vi "MTDC_Prototype.vi"() -> ()   [LabVIEW 2025]
uses:
  Desktop/STM-Auto-Project/QMH CTLS/Scan_Params (QMH).ctl
  <instrlib>/SMS LabVIEW Drivers/Source Code/Public/PSU Status.ctl
  Desktop/STM-Auto-Project/QMH CTLS/Sweeper.ctl
  <instrlib>/SMS LabVIEW Drivers/Source Code/Cryogenic Ltd SMSXXX.lvlib
  Downloads/OneDrive_2025-09-03/Instrument Controls/Temp Cntrl.ctl
  Desktop/Magnetic Drift Correction/XY_Coords(Final).ctl
panel:
  out "Translation (m)":T1
  out "Final coordinates (m)":cluster{"Xc":sgl, "Yc":sgl} {"Yc" format="%.4p"; "Xc" format="%.4p"}
  out "Initial coordinates (m)":cluster{"Xc":sgl, "Yc":sgl} {"Yc" format="%.4p"; "Xc" format="%.4p"}
  out "Temp. Array":dbl[](array[numeric])
  out "Current Temp":dbl format="%#.5f"
  out "Current MID (T)":dbl
  out "Output (T)":dbl
  in  "P-Mode Ramp Rate (A/s)":dbl=0.02
  out "Initial MID (T)":dbl
  in  "Serial Configuration":T2={"Baud Rate"=57600, "Parity"=1, "Data Bits"=7, "Stop Bits"=10, "Flow Control"=0}
  in  "Field and Temp Range":T3={"VISA (Magnet)"="COM4", "Fields(T)"=[], "Temps(K)"=[], "VISA (Temp) "="COM1", "Port number (3364)"=3364}
  in  "Lead- Mode Ramp Rate (A/s)":dbl=0.02
  out "Errors":errorcluster[](array[cluster])
  out "Current Index":i32
  in  "stop":bool
  in  "Start":bool
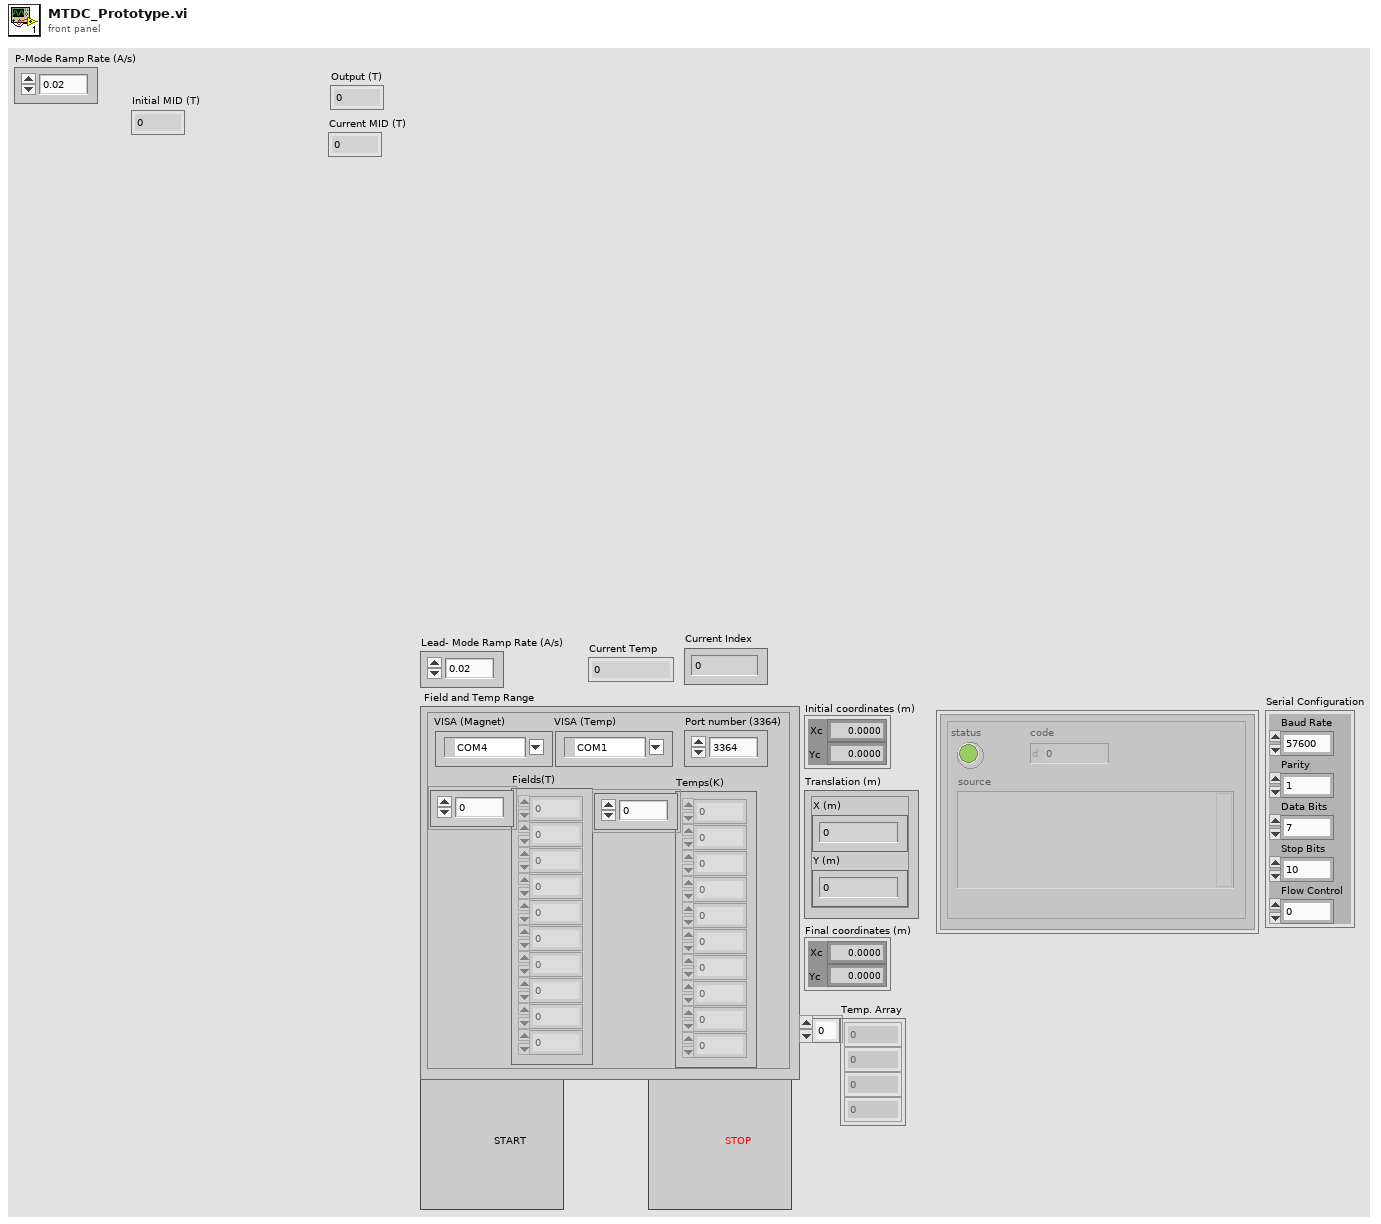
[diagram p1: front panel]
types:
  T1 = typedef "XY_Coords(Final).ctl" = cluster{"X (m)":dbl, "Y (m)":dbl}
  T2 = cluster{"Baud Rate":u32, "Parity":u16, "Data Bits":u16, "Stop Bits":u16, "Flow Control":u16}
  T3 = cluster{"VISA (Magnet)":refnum<visa-resource-name>, "Fields(T)":dbl[], "Temps(K)":dbl[], "VISA (Temp) ":refnum<visa-resource-name>, "Port number (3364)":u32}
  T4 = enum16{"1. INIT MAG", "2. MAG ON", "3. MAG_STAB", "4. MAG IDLE", "5. PREP NEXT FIELD", "6. APPLY NEXT FIELD", "7. PREP OFF", "8. MAG OFF (Reset)"}
  T5 = enum16{"1. BIAS", "2. INIT_SCAN", "3. SCAN_IDLE", "4. INTER_SCAN", "5. NEW_COORDS_&_FRAME", "6. FINAL_SCAN", "7. POLL BIAS ", "8. Z-CONT.", "9. STOP"}
  T6 = typedef "Temp Cntrl.ctl" = cluster{"Range (0:Off)":u16, "Manual Output (0.00 %)":dbl, "Rate (D) (0.0 %)":dbl, "Reset (I) (20.0)":dbl, "Gain (P) (50.0)":dbl, "Power Up Enable (F: Disable)":bool, "Max User Current (2.000)":dbl, "Heater Resistance (1:25 Ohms)":u16, "Max Current (0:User Specified)":u16, "Heater Out Display (1:Current)":u16, "Mode (0:Off)":u16, "Input (0:None)":u16, "Target Temp (K)":dbl, "Serial Configuration":cluster{"Baud Rate":u32, "Parity":u16, "Data Bits":u16, "Stop Bits":u16, "Flow Control":u16}, "VISA resource name":refnum<visa-resource-name>, "Configure Control Parameters (0: Configure)":u16, "Enable Setpoint (F:Disable)":bool, "Input (0:A)":u16, "Data Source (0:Kelvin)":u16, "Output's Control Loop (1:1)":u16, "STND DEV Threshold ":dbl, "Mean Tolerance ":dbl, "Current State":enum16{"1. INIT TEMP", "2. TC ON", "3. POLL_TEMPS", "4. TEMP_STAB", "5. TC IDLE", "6. APPLY NEXT TEMP", "7. TC OFF (Reset)"}}
  T7 = enum16{"NO CHANGE", "SET TEMP & FIELD", "SWEEP IDLE", "NEXT TEMP & FIELD", "SWEEP DONE"}
  T8 = typedef "Sweeper.ctl" = cluster{"Temps(K)":dbl[], "Fields(T)":dbl[], "Sweep States":enum16{"NO CHANGE", "SET TEMP & FIELD", "SWEEP IDLE", "NEXT TEMP & FIELD", "SWEEP DONE"}}
  T9 = enum16{"1. INIT TEMP", "2. TC ON", "3. POLL_TEMPS", "4. TEMP_STAB", "5. TC IDLE", "6. APPLY NEXT TEMP", "7. TC OFF (Reset)"}
  T10 = typedef "PSU Status.ctl" = cluster{"Ramp Target":enum16{"ZERO", "MID", "MAX"}, "Pause":bool, "Switch Heater":bool, "Persistent Field":dbl, "Persistent Current":dbl, "Tesla":bool, "Output (T)":dbl, "Output (A)":dbl, "X Trip":enum16{"DISABLED", "ENABLED", "ACTIVE"}, "Ramp Rate (A/s)":dbl, "V Limit (V)":dbl, "Heater Voltage":dbl, "MAX Setpoint (A)":dbl, "MAX Setpoint (T)":dbl, "MID Setpoint (A)":dbl, "MID Setpoint (T)":dbl, "Lock":bool, "Field Constant":dbl, "Remote":bool, "Direction":enum16{"POSITIVE", "NEGATIVE", "OPEN", "UNIPOLAR"}, "Helium Level":u16, "Quench !":bool, "Voltage":dbl, "V Limit !":bool, "Ramping":bool, "At Target":bool, "Trip Field":dbl, "Trip Current":dbl, "Current State":enum16{"1. INIT MAG", "2. MAG ON", "3. MAG_STAB", "4. MAG IDLE", "5. PREP NEXT FIELD", "6. APPLY NEXT FIELD", "7. PREP OFF", "8. MAG OFF (Reset)"}, "MAG Reference":refnum<visa-resource-name>}
  T11 = typedef "Scan_Params (QMH).ctl" = cluster{"Setpoint (I)":dbl[], "Bias (V)":dbl[], "Number of scans":u8, "Port number (3364)":u32, "Avoid zero threshold (V)":dbl, "Current State":enum16{"1. BIAS", "2. INIT_SCAN", "3. SCAN_IDLE", "4. INTER_SCAN", "5. NEW_COORDS_&_FRAME", "6. FINAL_SCAN", "7. POLL BIAS ", "8. Z-CONT.", "9. STOP"}}
  T12 = enum16{"RAMP TO ZERO", "RAMP TO MID", "RAMP TO MAX"}
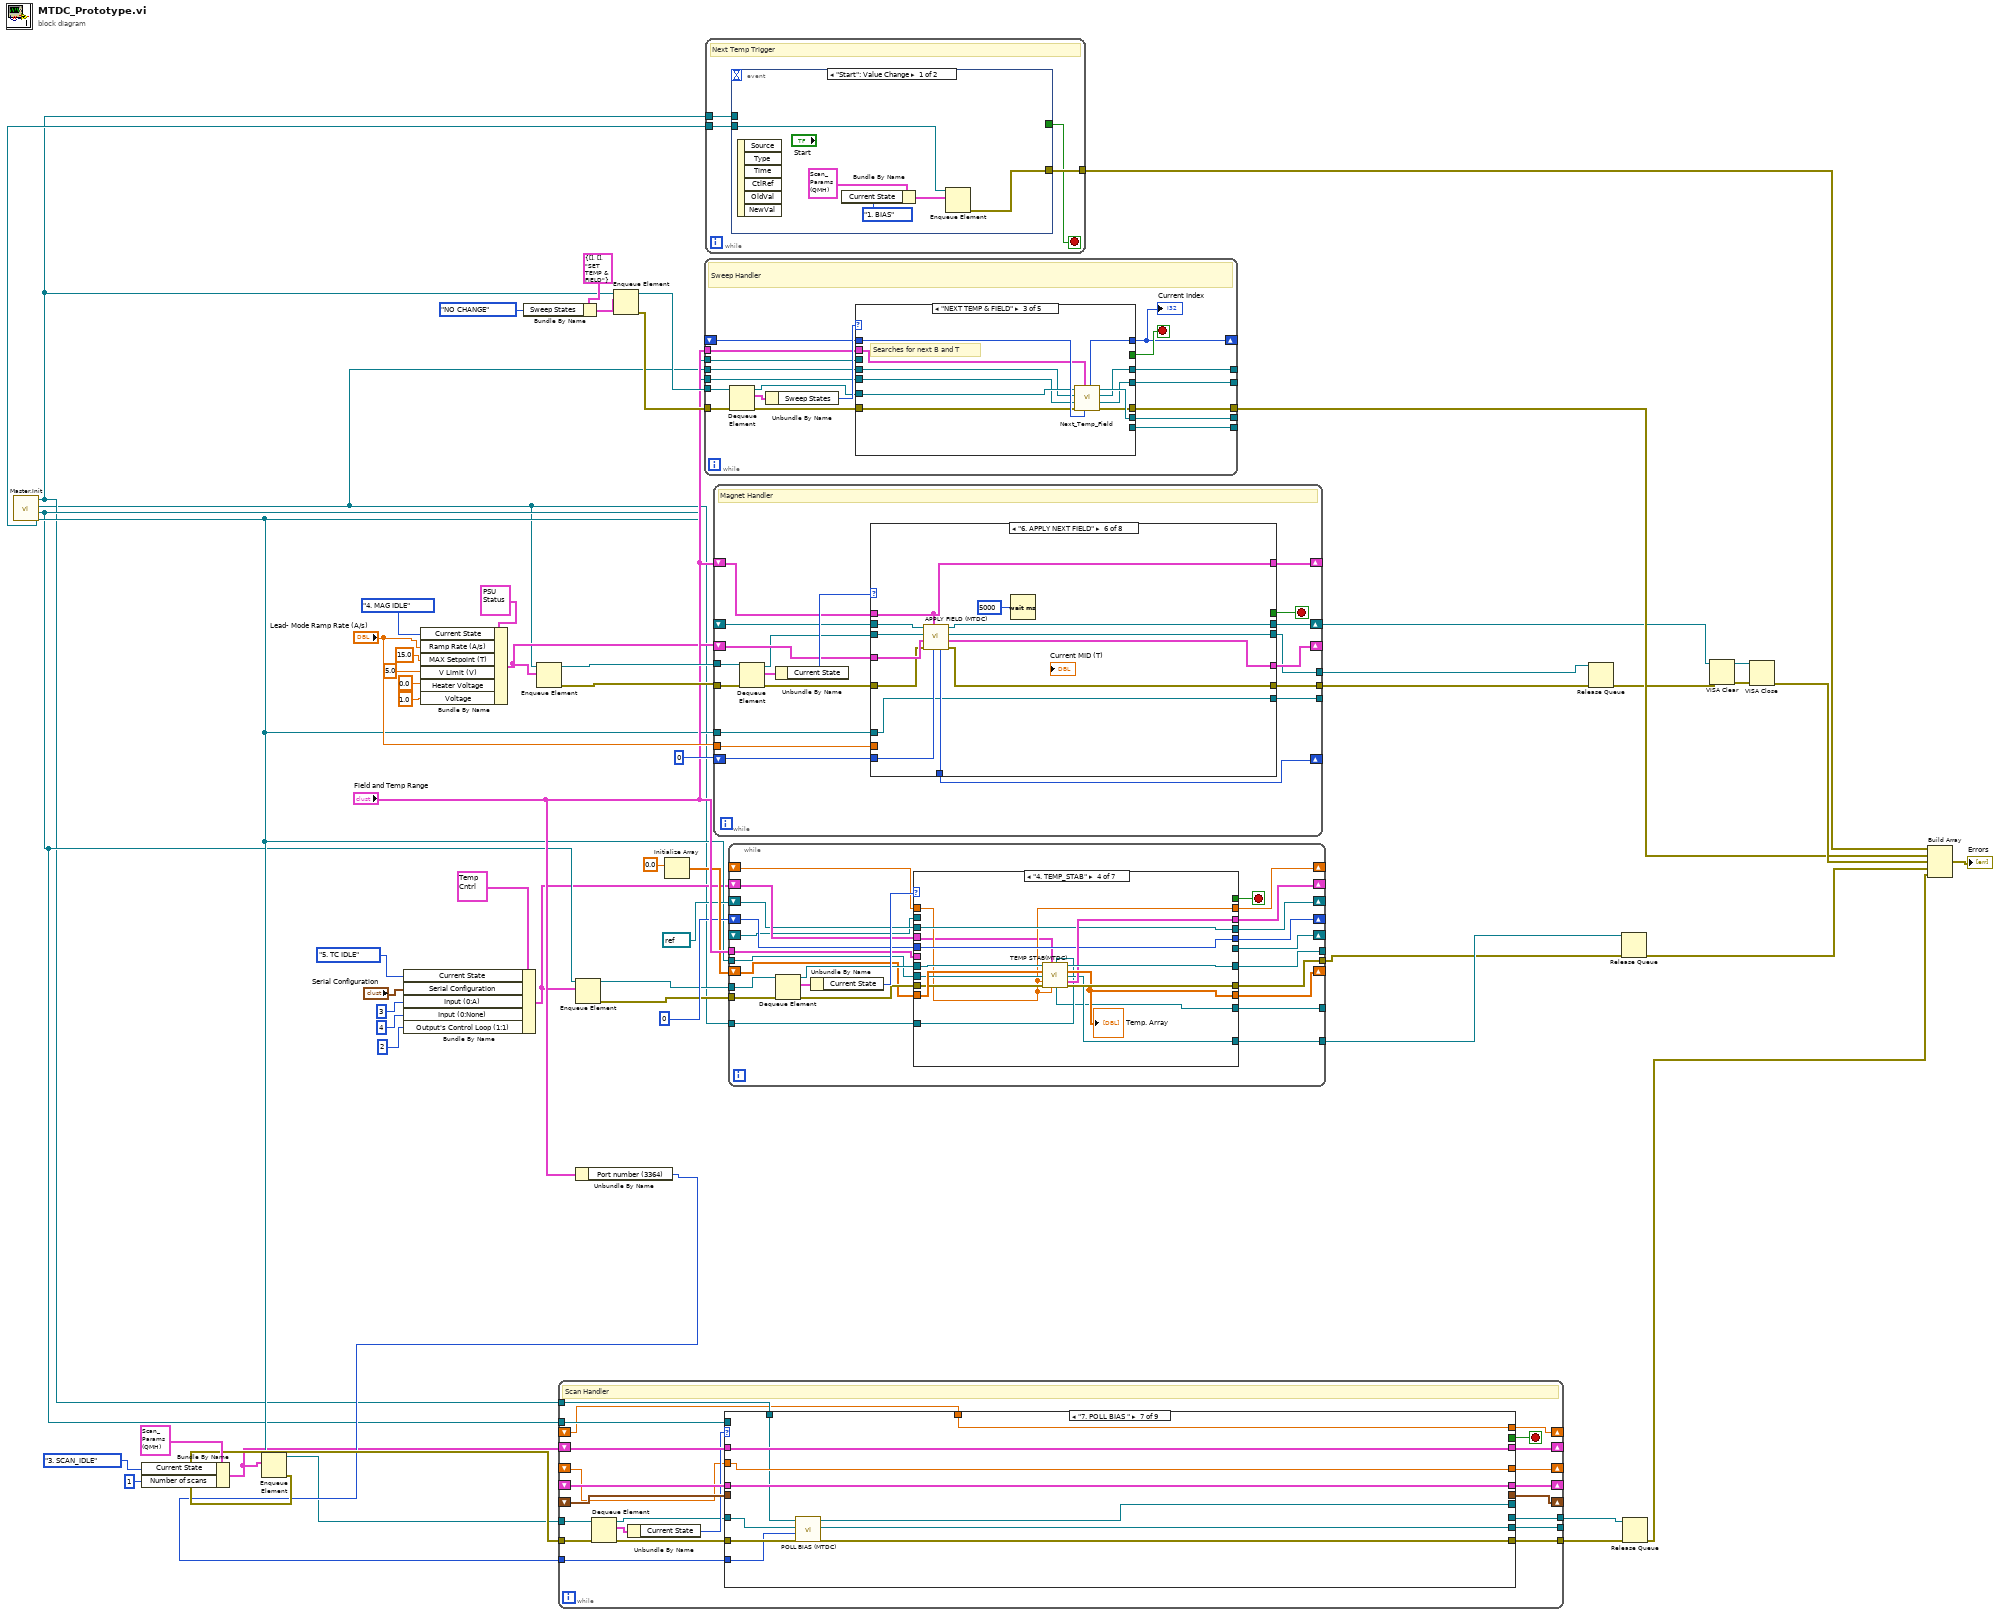
[diagram p0: block diagram]
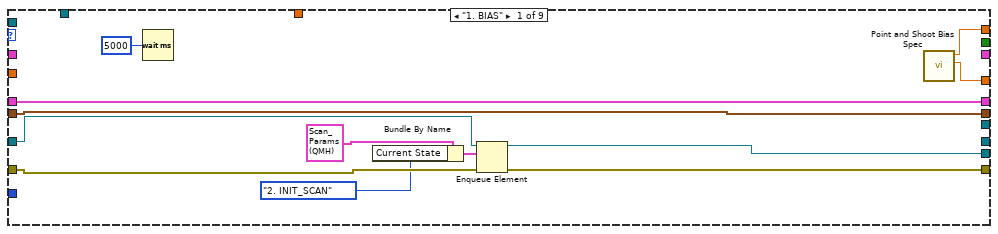
[diagram p2: hidden frame]
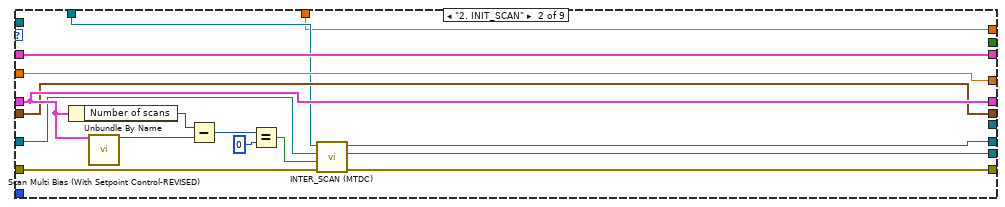
[diagram p3: hidden frame]
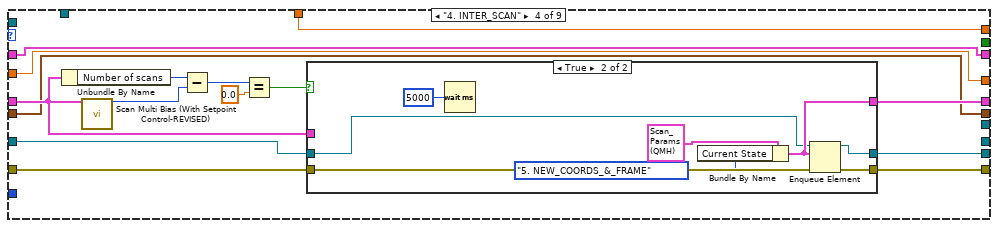
[diagram p5: hidden frame]
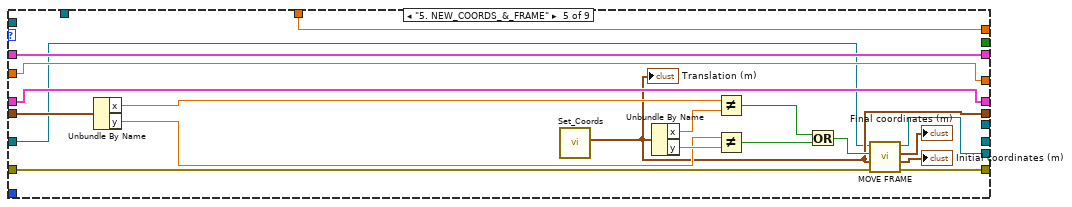
[diagram p7: hidden frame]
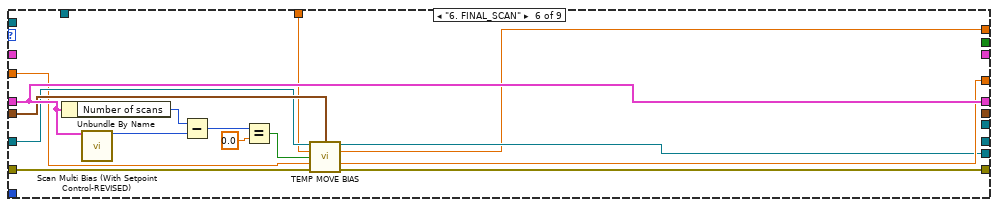
[diagram p8: hidden frame]
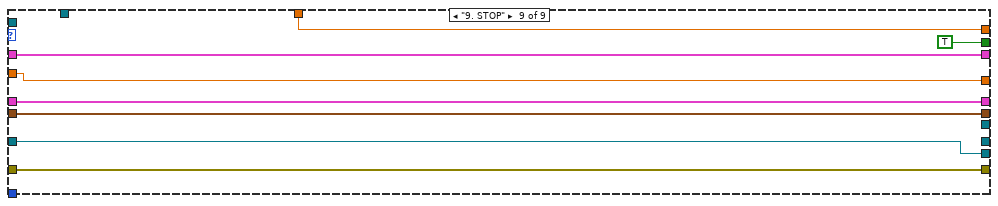
[diagram p10: hidden frame]
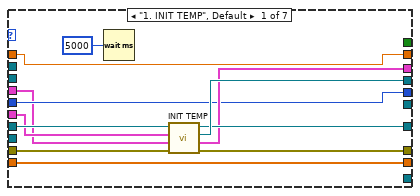
[diagram p11: hidden frame]
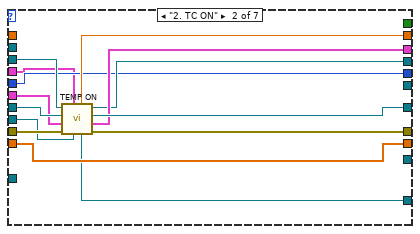
[diagram p12: hidden frame]
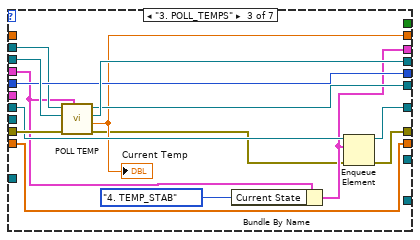
[diagram p13: hidden frame]
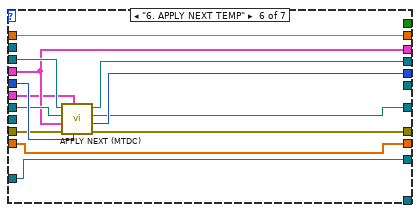
[diagram p15: hidden frame]
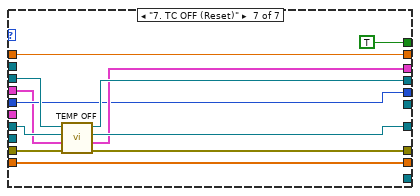
[diagram p16: hidden frame]
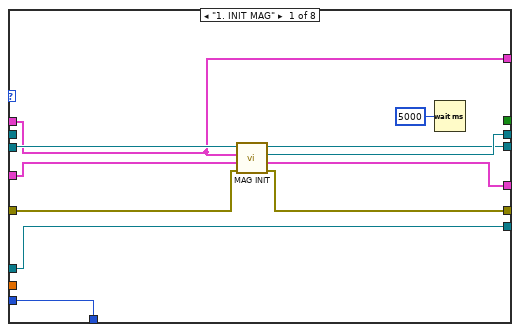
[diagram p17: hidden frame]
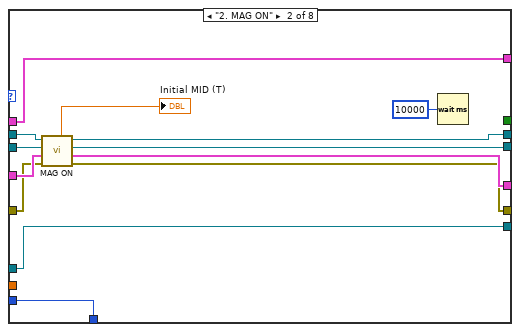
[diagram p18: hidden frame]
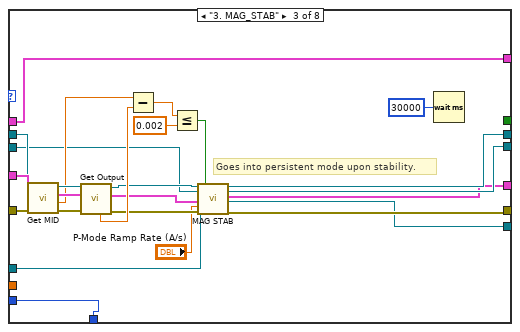
[diagram p19: hidden frame]
diagram:
  n1 = call "Master.Init.vi"() -> ("ScanQ"=w17:refnum<queue>, "TempQ"=w14:refnum<queue>, "MagQ"=w1:refnum<queue>, "SweepQ"=w2:refnum<queue>)  [unwired: 8 in]
  n2 = Bundle By Name(cluster=T11 {"Setpoint (I)"=[], "Bias (V)"=[], "Number of scans"=1, "Port number (3364)"=3364, "Avoid zero threshold (V)"=0.004999999888241291, "Current State"=enum."1. BIAS"} ("element"), "Current State"=T5."3. SCAN_IDLE", "Number of scans"=u8 1) -> (w5:T11)
  n3 = Enqueue Element(queue=w17, element=w5) -> (queue out=w16:refnum<queue>, error out=w19:errorcluster)  [unwired: 2 in, 1 out]
  n4 = Bundle By Name(cluster=T6 {"Range (0:Off)"=0, "Manual Output (0.00 %)"=0.0, "Rate (D) (0.0 %)"=0.0, "Reset (I) (20.0)"=20.0, "Gain (P) (50.0)"=50.0, "Power Up Enable (F: Disable)"=FALSE, "Max User Current (2.000)"=2.0, "Heater Resistance (1:25 Ohms)"=1, "Max Current (0:User Specified)"=0, "Heater Out Display (1:Current)"=1, "Mode (0:Off)"=1, "Input (0:None)"=4, "Target Temp (K)"=5.0, "Serial Configuration"={"Baud Rate"=57600, "Parity"=1, "Data Bits"=7, "Stop Bits"=10, "Flow Control"=0}, "VISA resource name"="", "Configure Control Parameters (0: Configure)"=0, "Enable Setpoint (F:Disable)"=FALSE, "Input (0:A)"=3, "Data Source (0:Kelvin)"=0, "Output's Control Loop (1:1)"=2, "STND DEV Threshold "=0.1, "Mean Tolerance "=0.02, "Current State"=enum."1. INIT TEMP"} ("element"), "Current State"=T9."5. TC IDLE", "Serial Configuration"="Serial Configuration", "Input (0:A)"=u16 3, "Input (0:None)"=u16 4, "Output's Control Loop (1:1)"=u16 2) -> (w6:T6)
  n5 = Bundle By Name(cluster=T10 {"Ramp Target"=enum."ZERO", "Pause"=FALSE, "Switch Heater"=FALSE, "Persistent Field"=0.0, "Persistent Current"=0.0, "Tesla"=FALSE, "Output (T)"=0.0, "Output (A)"=0.0, "X Trip"=enum."DISABLED", "Ramp Rate (A/s)"=0.0, "V Limit (V)"=0.0, "Heater Voltage"=0.0, "MAX Setpoint (A)"=0.0, "MAX Setpoint (T)"=0.0, "MID Setpoint (A)"=0.0, "MID Setpoint (T)"=0.0, "Lock"=FALSE, "Field Constant"=0.0, "Remote"=FALSE, "Direction"=enum."POSITIVE", "Helium Level"=0, "Quench !"=FALSE, "Voltage"=0.0, "V Limit !"=FALSE, "Ramping"=FALSE, "At Target"=FALSE, "Trip Field"=0.0, "Trip Current"=0.0, "Current State"=enum."1. INIT MAG", "MAG Reference"="COM4"} ("PSU Status In"), "Current State"=T4."4. MAG IDLE", "Ramp Rate (A/s)"="Lead- Mode Ramp Rate (A/s)", "MAX Setpoint (T)"=15.0, "V Limit (V)"=5.0, "Heater Voltage"=0.0, "Voltage"=1.0) -> (w7:T10)
  n6 = Bundle By Name(cluster=T8 {"Temps(K)"=[], "Fields(T)"=[], "Sweep States"=enum."SET TEMP & FIELD"} ("Temp and Field Range"), "Sweep States"=T7."NO CHANGE") -> (w40:T8)
  n7 = Enqueue Element(queue=w1, element=w7) -> (queue out=w35:refnum<queue>, error out=w36:errorcluster)  [unwired: 2 in, 1 out]
  n8 = Enqueue Element(queue=w14, element=w6) -> (queue out=w23:refnum<queue>, error out=w22:errorcluster)  [unwired: 2 in, 1 out]
  n9 = Unbundle By Name("Field and Temp Range") -> ("Port number (3364)"=w18:u32)
  n10 = while {
    tunnel: w19 -> [w74]
    shift-right: [w79] -> _
    shift-left: _ -> [w80]
    shift-right: [w78] -> _
    shift-left: _ -> [w77]
    tunnel: [w75] -> w20
    tunnel: [w72] -> w21
    shift-right: [w70] -> _
    shift-left: w5 -> [w71]
    tunnel: w16 -> [w69]
    shift-right: [w66] -> _
    shift-left: _ -> [w65]
    tunnel: [w64] -> _
    tunnel: w18 -> [w60]
    tunnel: w14 -> [w62]
    tunnel: w2 -> [w61]
    shift-right: [w58] -> _
    shift-left: _ -> [w59]
    stop <- w76 stop-if-true
    # "Scan Handler"
    n11 = Dequeue Element(queue=w69, error in (no error)=w74) -> (queue out=w63:refnum<queue>, element=w67:T11, error out=w73:errorcluster)  [unwired: 1 in, 1 out]
    n12 = Unbundle By Name(w67) -> ("Current State"=w68:T5)
    n13 = case shown="\"7. POLL BIAS \"" w68 {
      tunnel: w80 -> [w92 w105 w113 w123 w159 w171 w182 w190 w199]
      tunnel: w73 -> [w88 w99 _ w120 w149 w168 w181 w192 w200]
      tunnel: [w92 w105 w113 w124 w159 w171 w182 w190 w199] -> w79
      tunnel: [w91 w103 w114 w122 w146 _ _ w189 w198] -> w78
      tunnel: w77 -> [w91 w103 w114 w122 w151 w166 _ w189 w198]
      tunnel: [_ _ _ _ _ _ _ _ TRUE] -> w76
      tunnel: [w89 w95 _ w121 w150 w167 w179 w192 w200] -> w75
      tunnel: [_ w98 _ _ _ _ _ _ _] -> w72
      tunnel: w71 -> [_ w102 w112 w119 w145 _ w185 w187 w197]
      tunnel: [_ w102 w112 w119 w145 _ w185 w187 w197] -> w70
      tunnel: [w85 w101 w111 w118 w144 w163 w184 w188 w196] -> w66
      tunnel: w65 -> [_ w101 w111 w118 w144 w164 w184 w188 w196]
      tunnel: [w83 w97 w110 w116 w142 w162 w180 w193 w195] -> w64
      tunnel: w63 -> [w84 w96 w110 w117 w143 w165 w183 w193 w195]
      tunnel: w62 -> [_ _ _ _ _ _ _ _ _]
      tunnel: w61 -> [_ w94 _ _ _ _ w178 w191 _]
      tunnel: [_ _ _ _ _ _ w177 w191 _] -> _
      tunnel: w60 -> [_ _ _ _ _ _ w176 _ _]
      tunnel: w59 -> [_ w93 w109 w115 w141 w161 w175 w186 w194]
      tunnel: [w81 w93 w109 w115 w141 w160 w175 w186 w194] -> w58
      frame "1. BIAS" {
        n14 = Wait (ms)(milliseconds to wait=u32 5000) -> ()  [unwired: 1 out]
        n15 = Bundle By Name(cluster=T11 {"Setpoint (I)"=[], "Bias (V)"=[], "Number of scans"=1, "Port number (3364)"=3364, "Avoid zero threshold (V)"=0.004999999888241291, "Current State"=enum."1. BIAS"} ("element"), "Current State"=T5."2. INIT_SCAN") -> (w86:T11)
        n16 = Enqueue Element(queue=w84, element=w86, error in (no error)=w88) -> (queue out=w83:refnum<queue>, error out=w89:errorcluster)  [unwired: 1 in, 1 out]
        n17 = call "Point and Shoot Bias Spec.vi"() -> ("Initial Y (m)"=w85:dbl, "Inital X (m)"=w81:dbl)  [unwired: 10 in]
      }
      frame "2. INIT_SCAN" {
        n18 = Unbundle By Name(w105) -> ("Number of scans"=w104:u8)
        n19 = call "Scan Multi Bias (With Setpoint Control-REVISED).vi"("Scan Parameters"=w105) -> ("Scan"=w106:u8)  [unwired: 13 in, 1 out]
        n20 = Subtract(x=w104, y=w106) -> (x-y=w108:u8)
        n21 = Equal?(x=w108, y=u8 0) -> (x = y?=w100:bool)
        n22 = call "INTER_SCAN (MTDC).vi"("error in (no error)"=w99, "Boolean"=w100, "ScanQ in"=w96, "SweepQ 2"=w94) -> ("error out"=w95:errorcluster, "ScanQ out"=w97:refnum<queue>, "SweepQ"=w98:refnum<queue>)  [unwired: 5 in]
      }
      frame "3. SCAN_IDLE" {
      }
      frame "4. INTER_SCAN" {
        n23 = Unbundle By Name(w123) -> ("Number of scans"=w125:u8)
        n24 = call "Scan Multi Bias (With Setpoint Control-REVISED).vi"("Scan Parameters"=w123) -> ("Scan"=w126:u8)  [unwired: 13 in, 1 out]
        n25 = Subtract(x=w125, y=w126) -> (x-y=w128:u8)
        n26 = Equal?(x=w128, y=0.0) -> (x = y?=w127:bool)
        n27 = case shown="True" w127 {
          tunnel: [w132 w136] -> w124
          tunnel: w123 -> [w132 _]
          tunnel: [w131 w139] -> w121
          tunnel: w120 -> [w131 w138]
          tunnel: w117 -> [w130 w135]
          tunnel: [w130 w134] -> w116
          frame False {
          }
          frame True {
            n28 = Wait (ms)(milliseconds to wait=u32 5000) -> ()  [unwired: 1 out]
            n29 = Bundle By Name(cluster=T11 {"Setpoint (I)"=[], "Bias (V)"=[], "Number of scans"=1, "Port number (3364)"=3364, "Avoid zero threshold (V)"=0.004999999888241291, "Current State"=enum."2. INIT_SCAN"} ("element"), "Current State"=T5."5. NEW_COORDS_&_FRAME") -> (w136:T11)
            n30 = Enqueue Element(queue=w135, element=w136, error in (no error)=w138) -> (queue out=w134:refnum<queue>, error out=w139:errorcluster)  [unwired: 1 in, 1 out]
          }
        }
      }
      frame "5. NEW_COORDS_&_FRAME" {
        n31 = Unbundle By Name(w151) -> ("x"=w153:dbl, "y"=w152:dbl)
        n32 = call "Set_Coords.vi"() -> ("return value"=w146:cluster{"x":dbl, "y":dbl})  [unwired: 10 in, 1 out]
        "Translation (m)" <- w146
        n33 = Unbundle By Name(w146) -> ("x"=w156:dbl, "y"=w155:dbl)
        n34 = Not Equal?(x=w153, y=w156) -> (x != y?=w158:bool)
        n35 = Not Equal?(x=w152, y=w155) -> (x != y?=w157:bool)
        n36 = Or(x=w158, y=w157) -> (x .or. y?=w154:bool)
        n37 = call "MOVE FRAME.vi"("error in (no error)"=w149, "return value"=w146, "Boolean"=w154, "Queue in"=w143) -> ("error out"=w150:errorcluster, "Initial coordinates (m)"=→"Initial coordinates (m)":cluster{"Xc":sgl, "Yc":sgl}, "Final coordinates (m)"=→"Final coordinates (m)":cluster{"Xc":sgl, "Yc":sgl}, "Queue out"=w142:refnum<queue>)  [unwired: 4 in]
      }
      frame "6. FINAL_SCAN" {
        n38 = Unbundle By Name(w171) -> ("Number of scans"=w170:u8)
        n39 = call "Scan Multi Bias (With Setpoint Control-REVISED).vi"("Scan Parameters"=w171) -> ("Scan"=w172:u8)  [unwired: 13 in, 1 out]
        n40 = Subtract(x=w170, y=w172) -> (x-y=w173:u8)
        n41 = Equal?(x=w173, y=0.0) -> (x = y?=w169:bool)
        n42 = call "TEMP MOVE BIAS.vi"("ScanQ in"=w165, "Translation"=w166, "x"=w161, "Boolean"=w169, "y"=w164, "error in (no error)"=w168) -> ("ScanQ out"=w162:refnum<queue>, "X (m)"=w160:sgl, "Y (m)"=w163:sgl, "error out"=w167:errorcluster)  [unwired: 6 in]
      }
      frame "7. POLL BIAS " {
        n43 = call "POLL BIAS (MTDC).vi"("error in (no error)"=w181, "Port number (3364)"=w176, "ScanQ in"=w183, "SweepQ in"=w178) -> ("error out"=w179:errorcluster, "ScanQ out"=w180:refnum<queue>, "SweepQ out"=w177:refnum<queue>)  [unwired: 5 in]
      }
      frame "8. Z-CONT." {
      }
      frame "9. STOP" {
      }
    }
  }
  n44 = Enqueue Element(queue=w2, element=w40) -> (queue out=w55:refnum<queue>, error out=w54:errorcluster)  [unwired: 2 in, 1 out]
  n45 = Initialize Array(0.0 ("element")) -> (w26:dbl[])  [unwired: 1 in]
  n46 = while {
    tunnel: w55 -> [w218]
    shift-right: [w203] -> _
    shift-left: _ -> [w216]
    tunnel: [w215] -> _
    tunnel: [w213] -> _
    tunnel: [w211] -> w51
    tunnel: w54 -> [w209]
    tunnel: "Field and Temp Range" -> [w208]
    tunnel: w17 -> [w207]
    tunnel: [w206] -> _
    tunnel: w14 -> [w205]
    tunnel: [w204] -> _
    tunnel: w1 -> [w202]
    stop <- w210 stop-if-true
    # "Sweep Handler"
    n47 = Dequeue Element(queue=w218, error in (no error)=w209) -> (queue out=w214:refnum<queue>, element=w217:T8, error out=w212:errorcluster)  [unwired: 1 in, 1 out]
    n48 = Unbundle By Name(w217) -> ("Sweep States"=w219:T7)
    n49 = case shown="\"NEXT TEMP & FIELD\"" w219 {
      tunnel: w216 -> [_ w232 w244 _ w259]
      tunnel: [_ w233 w240 w246 w256] -> w215
      tunnel: w214 -> [w224 w231 w242 w248 w260]
      tunnel: [_ w232 w243 _ w259] -> w203
      tunnel: [w223 w230 w241 w248 w260] -> w213
      tunnel: w212 -> [_ w229 w238 w249 w257]
      tunnel: [_ w228 w239 w249 w255] -> w211
      tunnel: [_ _ _ _ w258] -> w210
      tunnel: w208 -> [w221 _ w235 _ _]
      tunnel: w207 -> [w220 _ _ w247 w253]
      tunnel: [w222 _ _ w247 w254] -> w206
      tunnel: w205 -> [_ w226 w237 w245 w252]
      tunnel: [_ w227 w234 w245 w251] -> w204
      tunnel: w202 -> [_ w225 w236 w246 w250]
      frame "NO CHANGE" {
        # "If no change, will just scan/bias"
        n50 = call "No_Change.vi"("Field and Temp Range"=w221, "ScanQ in"=w220, "Queue in"=w224) -> ("ScanQ out"=w222:refnum<queue>, "Queue out"=w223:refnum<queue>)  [unwired: 7 in]
      }
      frame "SET TEMP & FIELD" {
        # "Inits Mag and TC"
        n51 = call "Set_Temp_Field.vi"("error in (no error)"=w229, "TempQ In"=w226, "MagQ in"=w225, "Queue in"=w231) -> ("error out"=w228:errorcluster, "TempQ out"=w227:refnum<queue>, "MagQ out"=w233:refnum<queue>, "Queue out"=w230:refnum<queue>)  [unwired: 4 in]
      }
      frame "NEXT TEMP & FIELD" {
        # "Searches for next B and T"
        n52 = call "Next_Temp_Field.vi"("Numeric in"=w244, "Field and Temp Range"=w235, "error in (no error)"=w238, "TempQ in"=w237, "MagQ in"=w236, "Queue in"=w242) -> ("error out"=w239:errorcluster, "TempQ out"=w234:refnum<queue>, "MagQ out"=w240:refnum<queue>, "Queue out"=w241:refnum<queue>, "Numeric out"=w243:i32)  [unwired: 1 in]
      }
      frame "SWEEP IDLE" {
      }
      frame "SWEEP DONE" {
        # "Shutsdown instruments"
        n53 = call "Shutdown.vi"("error in (no error)"=w257, "TempQ in"=w252, "ScanQ in"=w253, "MaqQ in"=w250) -> ("error out"=w255:errorcluster, "TempQ Out"=w251:refnum<queue>, "ScanQ out"=w254:refnum<queue>, "Queue out"=w256:refnum<queue>, "Boolean"=w258:bool)  [unwired: 3 in]
      }
    }
    "Current Index" <- w203
  }
  n54 = while {
    tunnel: [w264] -> w52
    tunnel: w17 -> [w262]
    tunnel: w2 -> [w261]
    stop <- w263 stop-if-true
    # "Next Temp Trigger"
    n55 = event shown="[0] \"Start\": Value Change" {
      selector: _ -> [_ _]
      dyn-events: _ -> [_ _]
      timeout: _ -> [_ _]
      tunnel: [w269 w277] -> w264
      tunnel: [_ w275] -> w263
      tunnel: w262 -> [w267 _]
      tunnel: w261 -> [_ w270]
      event "Start": Value Change {
        n56 = event-data() -> ()  [unwired: 1 in, 6 out]
        n57 = Bundle By Name(cluster=T11 {"Setpoint (I)"=[], "Bias (V)"=[], "Number of scans"=1, "Port number (3364)"=3364, "Avoid zero threshold (V)"=0.004999999888241291, "Current State"=enum."1. BIAS"} ("element"), "Current State"=T5."1. BIAS") -> (w265:T11)
        n58 = Enqueue Element(queue=w267, element=w265) -> (error out=w269:errorcluster)  [unwired: 2 in, 2 out]
      }
      event "stop": Value Change {
        n59 = event-data() -> ()  [unwired: 1 in, 1 out]
        n60 = Bundle By Name(cluster=T8 {"Temps(K)"=[], "Fields(T)"=[], "Sweep States"=enum."SET TEMP & FIELD"} ("Temp and Field Range"), "Sweep States"=T7."SWEEP DONE") -> (w272:T8)
        n61 = Flush Queue(queue=w270) -> (queue out=w274:refnum<queue>)  [unwired: 1 in, 2 out]
        n62 = Enqueue Element At Opposite End(queue=w274, element=w272) -> (error out=w277:errorcluster)  [unwired: 2 in, 2 out]
        n63 = case shown="True" "stop" {
          tunnel: [FALSE ("stop 2") TRUE ("stop 2")] -> w275
          frame False {
          }
          frame True {
          }
        }
      }
    }
  }
  n64 = while {
    tunnel: [w295] -> w31
    shift-right: [w294] -> _
    shift-left: w7 -> [w297]
    shift-right: [w293] -> w30
    shift-left: _ -> [w292]
    tunnel: [w291] -> w32
    tunnel: w36 -> [w290]
    shift-right: [w284] -> _
    shift-left: 0 -> [w288]
    tunnel: "Lead- Mode Ramp Rate (A/s)" -> [w286]
    tunnel: w17 -> [w285]
    shift-right: [w282] -> _
    shift-left: "Field and Temp Range" -> [w289]
    tunnel: w35 -> [w281]
    tunnel: [w280] -> _
    stop <- w283 stop-if-true
    # "Magnet Handler"
    n65 = Dequeue Element(queue=w281, error in (no error)=w290) -> (queue out=w287:refnum<queue>, element=w299:T10, error out=w296:errorcluster)  [unwired: 1 in, 1 out]
    n66 = Unbundle By Name(w299) -> ("Current State"=w298:T4)
    n67 = case "MAG STATE MACHINE" shown="\"6. APPLY NEXT FIELD\"" w298 {
      tunnel: w297 -> [w306 w323 w347 w355 w365 w375 w401 w418]
      tunnel: w296 -> [w305 w321 w348 w354 _ w374 w400 w419]
      tunnel: [w309 w318 w330 w354 w362 w378 w383 w407] -> w295
      tunnel: [w307 w319 w331 w355 _ w371 w384 w410] -> w294
      tunnel: [w310 w320 w334 w353 w361 w372 w386 w411] -> w293
      tunnel: w292 -> [_ w322 w346 w353 w364 w376 w402 w420]
      tunnel: [w308 w317 w335 w350 w366 w379 w385 w409] -> w291
      tunnel: w289 -> [w301 w313 w327 w351 w358 w368 w381 w406]
      tunnel: w288 -> [w303 w314 w328 w352 w359 w373 w382 _]
      tunnel: w287 -> [w302 w312 w326 w350 w357 w369 _ w404]
      tunnel: w286 -> [_ _ _ _ w363 _ _ _]
      tunnel: w285 -> [w300 w311 w325 w349 w356 w367 w380 w405]
      tunnel: [w303 w314 w328 w352 w359 w370 w382 _] -> w284
      tunnel: [_ _ _ _ _ _ _ w408] -> w283
      tunnel: [w301 w313 w327 w351 w358 w368 w381 w406] -> w282
      tunnel: [w300 w311 w324 w349 w356 w367 w380 w405] -> w280
      frame "1. INIT MAG" {
        n68 = call "MAG INIT.vi"("error in (no error)"=w305, "PSU Status In"=w306, "Field and Temp Range"=w301, "Queue in"=w302) -> ("error out"=w309:errorcluster, "PSU Status Out"=w307:T10, "VISA Resource Name Out"=w310:refnum<visa-resource-name>, "Queue out"=w308:refnum<queue>)  [unwired: 4 in]
        n69 = Wait (ms)(milliseconds to wait=u32 5000) -> ()  [unwired: 1 out]
      }
      frame "2. MAG ON" {
        n70 = call "MAG ON.vi"("error in (no error)"=w321, "PSU Status In"=w323, "MagQ in"=w312, "VISA Refnum in"=w322) -> ("error out"=w318:errorcluster, "PSU Status Out"=w319:T10, "MagQ out"=w317:refnum<queue>, "VISA Refnum out"=w320:refnum<visa-resource-name>, "MID Setpoint (T)"=→"Initial MID (T)":dbl)  [unwired: 3 in]
        n71 = Wait (ms)(milliseconds to wait=u32 10000) -> ()  [unwired: 1 out]
      }
      frame "3. MAG_STAB" {
        # "Goes into persistent mode upon stability."
        n72 = call <instrlib>:"Get MID.vi"("Error in (no error)"=w348, "PSU Status In"=w347, "VISA Resource Name In"=w346) -> ("Error out"=w345:errorcluster, "MID Setpoint (T)"=w341:dbl, "PSU Status Out"=w344:T10, "VISA Resource Name Out"=w343:refnum<visa-resource-name>)  [unwired: 3 in, 2 out]
        n73 = call <instrlib>:"Get Output.vi"("Error in (no error)"=w345, "PSU Status In"=w344, "VISA Resource Name In"=w343) -> ("Error out"=w336:errorcluster, "PSU Status Out"=w337:T10, "VISA Resource Name Out"=w338:refnum<visa-resource-name>, "Output (T)"=w339:dbl)  [unwired: 3 in, 2 out]
        n74 = Subtract(x=w341, y=w339) -> (x-y=w340:dbl)
        n75 = Less Or Equal?(x=w340, y=0.002) -> (x <= y?=w333:bool)
        n76 = call "MAG STAB.vi"("VISA In"=w338, "MagQ"=w326, "ScanQ"=w325, "PSU Status In"=w337, "P-Mode Ramp Rate (A/s)"="P-Mode Ramp Rate (A/s)", "Error out"=w336, "Boolean"=w333) -> ("VISA Out"=w334:refnum<visa-resource-name>, "MagQ"=w335:refnum<queue>, "PSU Status Out"=w331:T10, "ScanQ out"=w324:refnum<queue>, "error out"=w330:errorcluster)  [unwired: 8 in]
        n77 = Wait (ms)(milliseconds to wait=u32 30000) -> ()  [unwired: 1 out]
      }
      frame "4. MAG IDLE" {
      }
      frame "5. PREP NEXT FIELD" {
        n78 = call "PREP FIELD.vi"("Numeric"=w359, "Lead- Mode Ramp Rate (A/s)"=w363, "PSU Status In"=w365, "MagQ in"=w357, "VISA Refnum in"=w364) -> ("error out"=w362:errorcluster, "Output (T)"=→"Output (T)":dbl, "MagQ out"=w366:refnum<queue>, "VISA Refnum out"=w361:refnum<visa-resource-name>)  [unwired: 3 in]
      }
      frame "6. APPLY NEXT FIELD" {
        n79 = call "APPLY FIELD (MTDC).vi"("Numeric in"=w373, "Field and Temp Range"=w368, "error in (no error)"=w374, "PSU Status In"=w375, "MagQ in"=w369, "VISA Refnum in"=w376) -> ("error out"=w378:errorcluster, "PSU Status Out"=w371:T10, "MagQ out"=w379:refnum<queue>, "VISA Refnum out"=w372:refnum<visa-resource-name>, "Numeric out"=w370:i32)  [unwired: 1 in]
        n80 = Wait (ms)(milliseconds to wait=u32 5000) -> ()  [unwired: 1 out]
      }
      frame "7. PREP OFF" {
        # "Assuming Heater is in off state to start."
        n81 = call <instrlib>:"Ramp.vi"("Error in (no error)"=w400, "Ramp Target"=T12."RAMP TO MID", "PSU Status In"=w401, "VISA Resource Name In"=w402) -> ("Error out"=w397:errorcluster, "PSU Status Out"=w398:T10, "VISA Resource Name Out"=w399:refnum<visa-resource-name>)  [unwired: 4 in, 1 out]
        n82 = call <instrlib>:"Get MID.vi"("Error in (no error)"=w397, "PSU Status In"=w398, "VISA Resource Name In"=w399) -> ("MID Setpoint (T)"=w391:dbl, "PSU Status Out"=w395:T10, "VISA Resource Name Out"=w396:refnum<visa-resource-name>)  [unwired: 3 in, 3 out]
        n83 = call <instrlib>:"Get Output.vi"("PSU Status In"=w395, "VISA Resource Name In"=w396) -> ("Error out"=w387:errorcluster, "PSU Status Out"=w388:T10, "VISA Resource Name Out"=w390:refnum<visa-resource-name>, "Output (T)"=w392:dbl)  [unwired: 4 in, 2 out]
        n84 = Subtract(x=w391, y=w392) -> (x-y=w394:dbl)
        n85 = Less Or Equal?(x=w394, y=0.002) -> (x <= y?=w389:bool)
        n86 = call "MAG PREP.vi"("VISA In"=w390, "Boolean"=w389, "PSU Status In"=w388, "Error In"=w387) -> ("VISA Out"=w386:refnum<visa-resource-name>, "MagQ"=w385:refnum<queue>, "PSU Status Out"=w384:T10, "error out"=w383:errorcluster)  [unwired: 8 in]
      }
      frame "8. MAG OFF (Reset)" {
        n87 = call <instrlib>:"Get Output.vi"("Error in (no error)"=w419, "PSU Status In"=w418, "VISA Resource Name In"=w420) -> ("Error out"=w413:errorcluster, "PSU Status Out"=w414:T10, "VISA Resource Name Out"=w415:refnum<visa-resource-name>, "Output (T)"=w417:dbl)  [unwired: 3 in, 2 out]
        n88 = Less Or Equal?(x=w417, y=0.001) -> (x <= y?=w412:bool)
        n89 = call "MAG OFF.vi"("VISA Resource Name Out"=w415, "MagQ"=w404, "Boolean"=w412, "PSU Status Out"=w414, "Error out"=w413) -> ("VISA Resource Name Out 2"=w411:refnum<visa-resource-name>, "MagQ 2"=w409:refnum<queue>, "Boolean 2"=w408:bool, "PSU Status Out 2"=w410:T10, "error out"=w407:errorcluster)  [unwired: 6 in]
      }
    }
  }
  n90 = while {
    tunnel: w23 -> [w446]
    tunnel: w22 -> [w445]
    shift-right: [w423] -> _
    shift-left: w6 -> [w442]
    tunnel: "Field and Temp Range" -> [w440]
    shift-right: [w439] -> _
    shift-left: refnum<visa-resource-name> refnum ("VISA Refnum out") -> [w435]
    tunnel: [w438] -> w28
    tunnel: [w436] -> _
    shift-right: [w431] -> _
    shift-left: _ -> [w434]
    shift-right: [w432] -> _
    shift-left: w26 -> [w433]
    tunnel: w17 -> [w430]
    tunnel: [w429] -> w29
    shift-right: [w427] -> _
    shift-left: 0 -> [w428]
    shift-right: [w425] -> _
    shift-left: _ -> [w424]
    tunnel: w1 -> [w422]
    tunnel: [w421] -> _
    stop <- w426 stop-if-true
    n91 = Dequeue Element(queue=w446, error in (no error)=w445) -> (queue out=w437:refnum<queue>, element=w444:T6, error out=w441:errorcluster)  [unwired: 1 in, 1 out]
    n92 = Unbundle By Name(w444) -> ("Current State"=w443:T9)
    n93 = case shown="\"4. TEMP_STAB\"" w443 {
      tunnel: w442 -> [w447 w459 w474 w490 w504 w513 w524]
      tunnel: w441 -> [w458 w467 w486 w500 w506 w519 w533]
      tunnel: w440 -> [w448 w460 _ _ _ w511 _]
      tunnel: [w457 w466 w485 w492 w507 w518 w532] -> w439
      tunnel: [w454 w470 w481 w498 w506 w515 w530] -> w438
      tunnel: w437 -> [w456 w472 w483 w501 w508 w517 w531]
      tunnel: [w455 w471 w482 w499 w508 w516 w529] -> w436
      tunnel: [w452 w469 w475 w496 w504 w513 w528] -> w423
      tunnel: w435 -> [_ w468 w487 w492 w507 w520 w534]
      tunnel: [w450 w465 w476 w491 w509 w514 w526] -> w431
      tunnel: w434 -> [w450 _ _ w491 w509 w514 w526]
      tunnel: w433 -> [w451 w464 w477 w502 w510 w523 w535]
      tunnel: [w451 w464 w477 w497 w510 w523 w535] -> w432
      tunnel: w430 -> [_ w462 _ w495 _ _ _]
      tunnel: [_ w461 _ w494 _ _ _] -> w429
      tunnel: w428 -> [w449 w463 w484 w493 w505 w522 w527]
      tunnel: [w449 w463 w484 w493 w505 w521 w527] -> w427
      tunnel: [_ _ _ _ _ _ TRUE] -> w426
      tunnel: [_ _ w480 _ _ _ _] -> w425
      tunnel: w424 -> [_ _ w478 _ _ _ _]
      tunnel: w422 -> [_ _ _ w489 w503 w512 _]
      tunnel: [_ _ _ w488 w503 w512 _] -> w421
      frame "1. INIT TEMP", Default {
        n94 = Wait (ms)(milliseconds to wait=u32 5000) -> ()  [unwired: 1 out]
        n95 = call "INIT TEMP.vi"("error in (no error)"=w458, "element"=w447, "Field and Temp Range"=w448, "Queue in"=w456) -> ("error out"=w454:errorcluster, "output cluster"=w452:T6, "VISA resource name out"=w457:refnum<visa-resource-name>, "Queue out"=w455:refnum<queue>)  [unwired: 4 in]
      }
      frame "2. TC ON" {
        n96 = call "TEMP ON.vi"("ScanQ in"=w462, "element in"=w459, "error in (no error)"=w467, "Field and Temp Range 2"=w460, "TempQ in"=w472, "VISA Refnum in"=w468) -> ("error out"=w470:errorcluster, "element out"=w469:T6, "TempQ out"=w471:refnum<queue>, "VISA Refnum out"=w466:refnum<visa-resource-name>, "ScanQ out"=w461:refnum<queue>, "Setpoint"=w465:dbl)
      }
      frame "3. POLL_TEMPS" {
        n97 = call "POLL TEMP.vi"("element"=w474, "error in (no error)"=w486, "VISA resource name in"=w487, "Queue in"=w478) -> ("error out"=w473:errorcluster, "Sensor Data"=w476:dbl, "VISA resource name out"=w485:refnum<visa-resource-name>, "Queue out"=w480:refnum<queue>)  [unwired: 4 in]
        "Current Temp" <- w476
        n98 = Bundle By Name(cluster=w474, "Current State"=T9."4. TEMP_STAB") -> (w475:T6)
        n99 = Enqueue Element(queue=w483, element=w475, error in (no error)=w473) -> (queue out=w482:refnum<queue>, error out=w481:errorcluster)  [unwired: 1 in, 1 out]
      }
      frame "4. TEMP_STAB" {
        n100 = call "TEMP STAB(MTDC).vi"("Queue in"=w501, "element in"=w490, "MagQ in"=w489, "Array in"=w502, "ScanQ In"=w495, "Setpoint"=w491, "error in (no error)"=w500, "element"=w491) -> ("Queue out"=w499:refnum<queue>, "Array out"=w497:dbl[], "ScanQ"=w494:refnum<queue>, "element out"=w496:T6, "MagQ out"=w488:refnum<queue>, "error out"=w498:errorcluster)  [unwired: 2 in]
        "Temp. Array" <- w497
      }
      frame "5. TC IDLE" {
      }
      frame "6. APPLY NEXT TEMP" {
        n101 = call "APPLY NEXT (MTDC).vi"("Numeric in"=w522, "Field and Temp Range 2"=w511, "error in (no error)"=w519, "element in"=w513, "TempQ in"=w517, "VISA Refnum in"=w520) -> ("error out"=w515:errorcluster, "Numeric out"=w521:i32, "TempQ out"=w516:refnum<queue>, "VISA Refnum out"=w518:refnum<visa-resource-name>)  [unwired: 2 in]
      }
      frame "7. TC OFF (Reset)" {
        n102 = call "TEMP OFF.vi"("error in (no error)"=w533, "element in"=w524, "TempQ in"=w531, "VISA Refnum in"=w534) -> ("error out"=w530:errorcluster, "element out"=w528:T6, "TempQ out"=w529:refnum<queue>, "VISA Refnum out"=w532:refnum<visa-resource-name>)  [unwired: 4 in]
      }
    }
  }
  n103 = Release Queue(queue=w32, error in (no error)=w31) -> (error out=w45:errorcluster)  [unwired: 1 in, 2 out]
  n104 = Release Queue(queue=w29, error in (no error)=w28) -> (error out=w39:errorcluster)  [unwired: 1 in, 2 out]
  n105 = Release Queue(queue=w21, error in (no error)=w20) -> (error out=w38:errorcluster)  [unwired: 1 in, 2 out]
  n106 = VISA Clear(VISA resource name=w30, error in (no error)=w45) -> (VISA resource name out=w44:refnum<visa-resource-name>, error out=w43:errorcluster)
  n107 = VISA Close(VISA resource name=w44, error in (no error)=w43) -> (error out=w57:errorcluster)
  n108 = Build Array(w52, w51, w57, w39, w38) -> (→"Errors":errorcluster[])
